vi "Intan_StreamData.vi"(0 "VISA resource name":refnum<visa-resource-name>, 1 "N data blocks to read":i32=1, 5 "refnum in":refnum<file>, 7 "stop":bool, 9 "Save to Disk":bool, 11 "error in":errorcluster, 12 "byte order":T2(ring)=enum."little-endian", 13 "DT_scale":dbl=0.01) -> (2 "Nbytes read":u32, 3 "Nchans1samp_array":u16[](array[numeric]), 4 "Intan Streaming Data  Chart":dbl[][](graph), 6 "path":path, 14 "iteration":i32, 15 "error out":errorcluster)   [LabVIEW 2011]
uses:
  <userlib>/Circular Buffer/Circular Buffer.lvlib
  <userlib>/Circular Buffer/Instance VIs/Circular Buffer(2D I16).vi
  <userlib>/Circular Buffer/Controls/Circular Buffer Operations.ctl
panel:
  out "cluster":T1
  in  "DisplayScale (uV/div)":u16(ring) items=["6400", "3200", "1600", "800", "400", "200", "100", "50", "25"]
  in  "offset factor":dbl=1.0
  out "timestamp":u32[](array[numeric])
  out "'IN' subarray (from INTAN)":u16[](array[numeric])
  in  "start stream (Teensy char)":string="s"
  out "Text response":string
  in  "pause stream (Teensy char)":string="p"
  in  "bytes per block":i32=72
  out "strlen":i32
  out "Nchans":i32
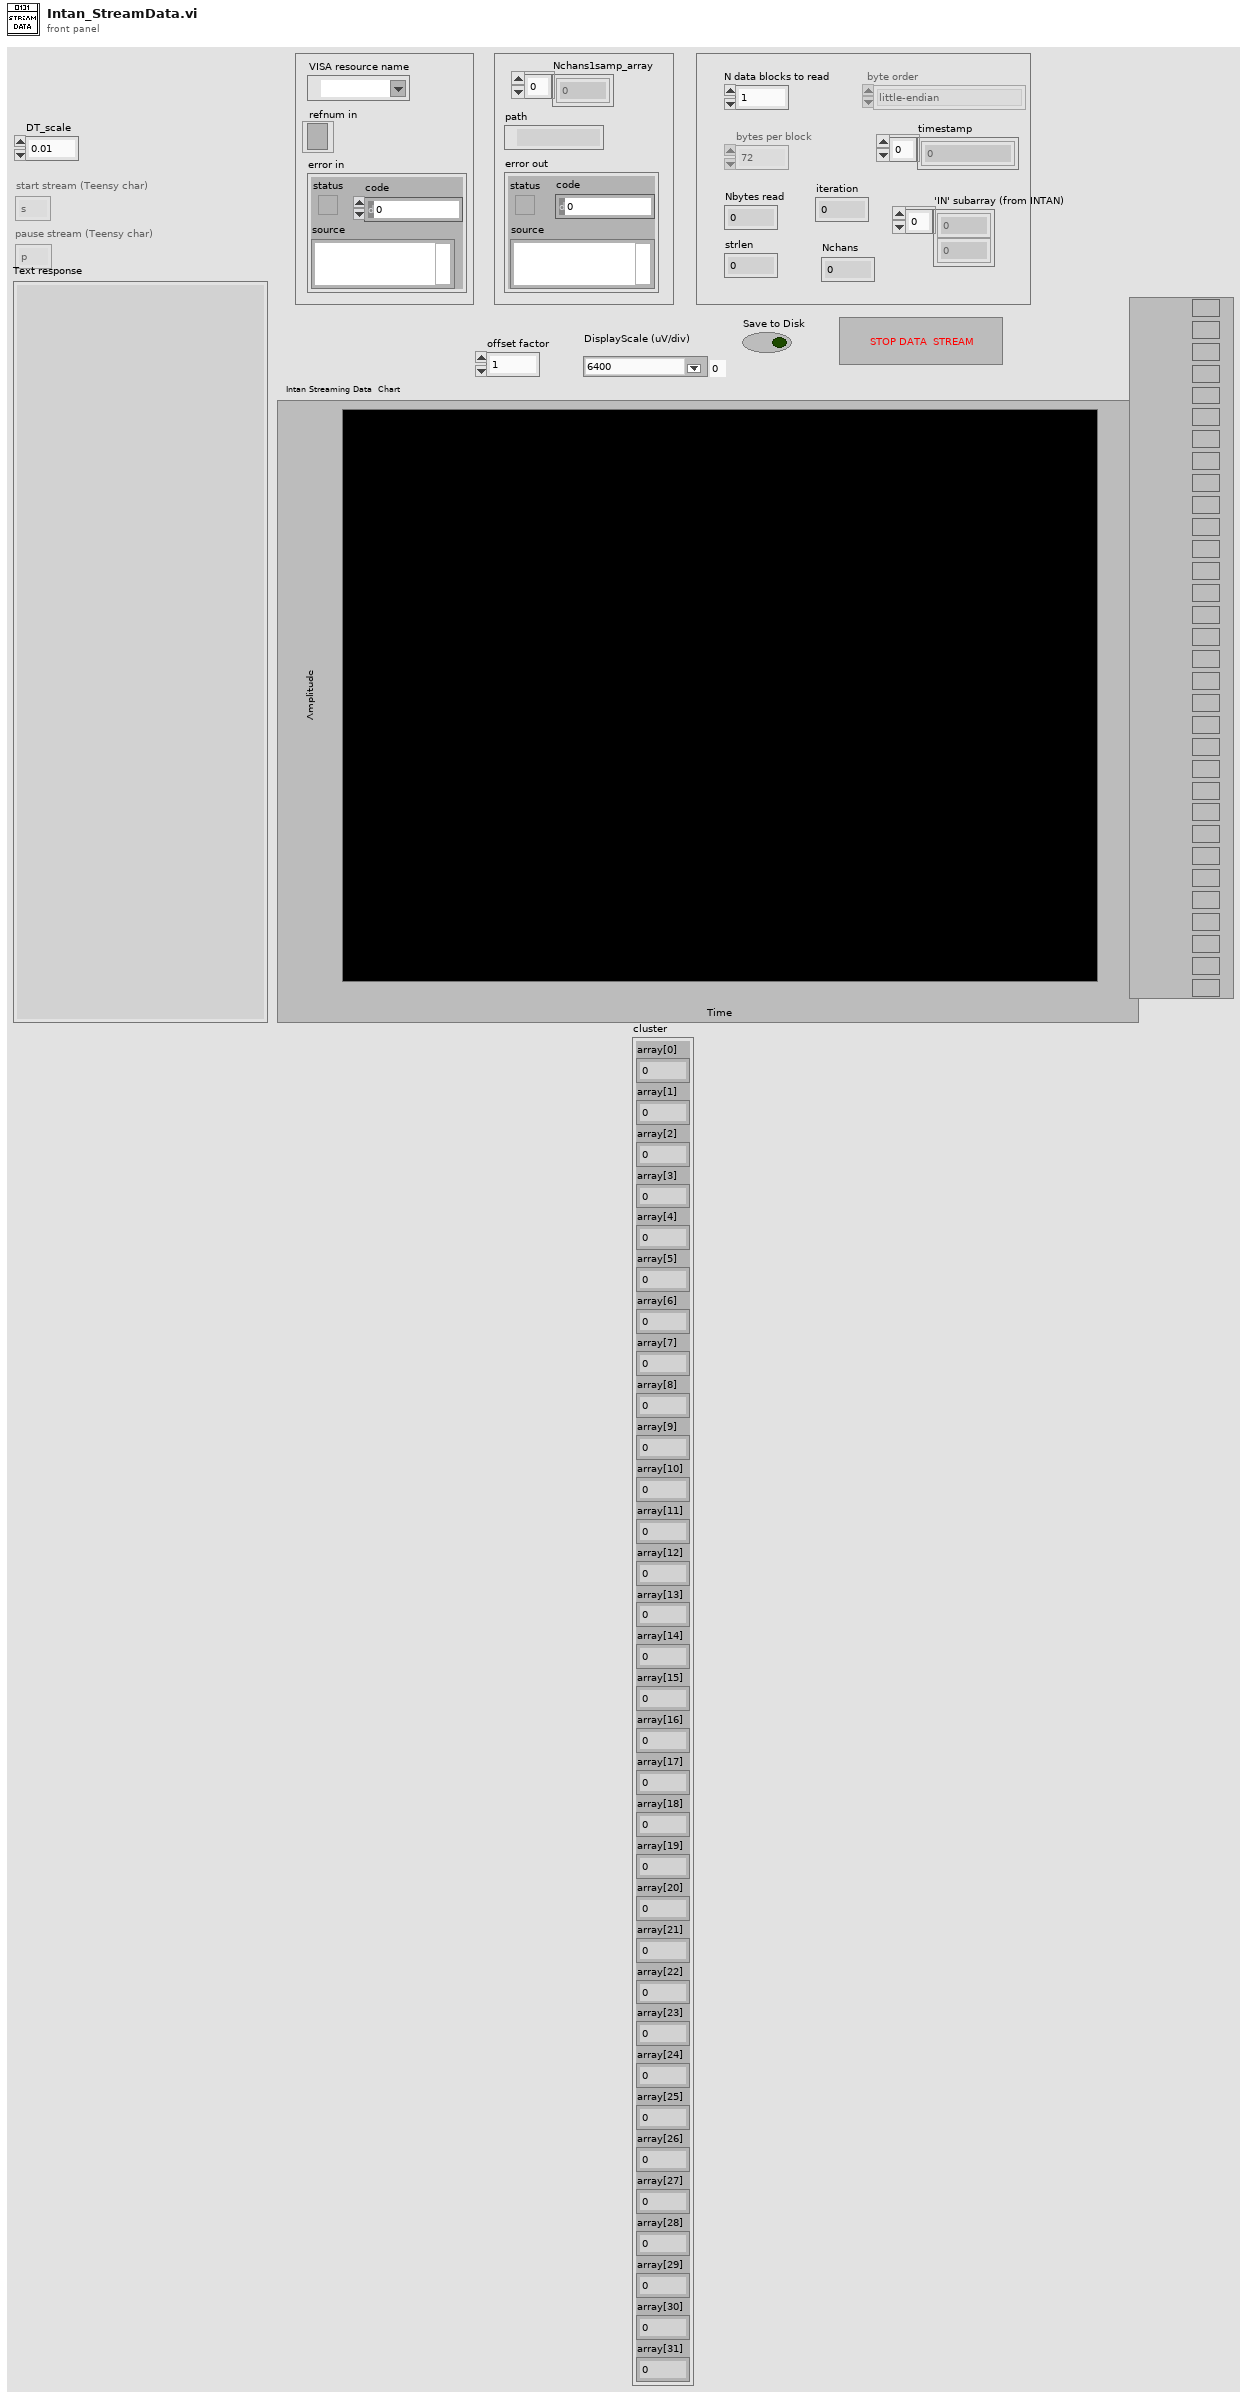
[diagram p1: front panel]
types:
  T1 = cluster{"array[0]":i32, "array[1]":i32, "array[2]":i32, "array[3]":i32, "array[4]":i32, "array[5]":i32, "array[6]":i32, "array[7]":i32, "array[8]":i32, "array[9]":i32, "array[10]":i32, "array[11]":i32, "array[12]":i32, "array[13]":i32, "array[14]":i32, "array[15]":i32, "array[16]":i32, "array[17]":i32, "array[18]":i32, "array[19]":i32, "array[20]":i32, "array[21]":i32, "array[22]":i32, "array[23]":i32, "array[24]":i32, "array[25]":i32, "array[26]":i32, "array[27]":i32, "array[28]":i32, "array[29]":i32, "array[30]":i32, "array[31]":i32}
  T2 = enum16{"big-endian, network order", "native, host order", "little-endian"}
  T3 = cluster{"Samples per Channel":u32, "Channels":u32}
  T4 = typedef "Circular Buffer.lvlib/Circular Buffer Operations.ctl" = enum16{"Initialize", "Get Backlog", "Write", "Read (continuous)", "Read (most recent)"}
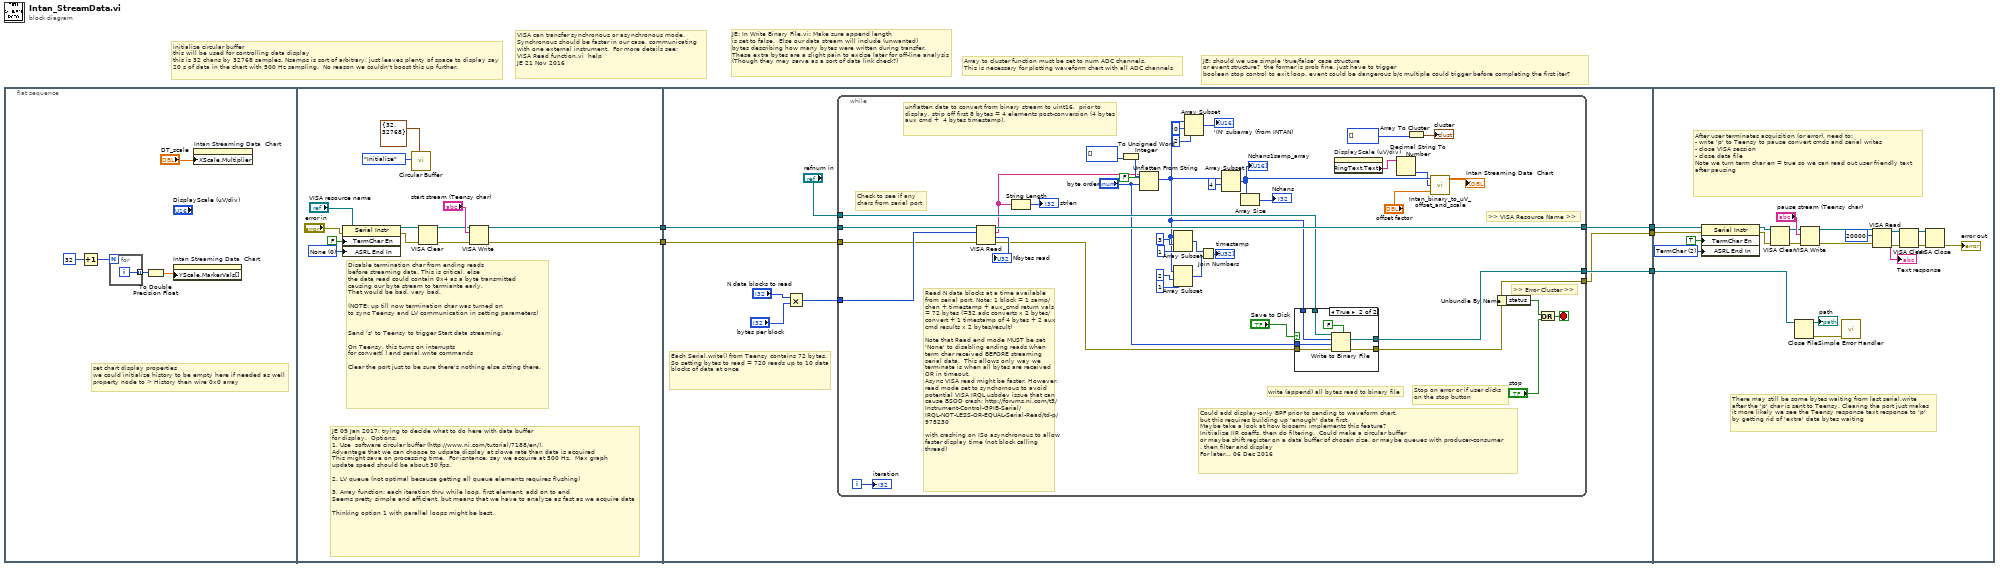
[diagram p0: block diagram]
diagram:
  # "initialize circular buffer\nthis will be used for controlling data display\nthis is 32 chans by 32768 samples. Nsamps is sort of arbitrary, just leaves plenty of space to display say\n20 s of data in the chart with 500 Hz sampling.  No reason we couldn't boost this up further."
  # "JE: should we use simple 'true/false' case structure\nor event structure?  the former is prob fine, just have to trigger\nboolean stop control to exit loop. event could be dangerous b/c multiple could trigger before completing the first iter?"
  # "Array to cluster function must be set to num ADC channels. \nThis is necessary for plotting waveform chart with all ADC channels"
  # "JE: In Write Binary File.vi: Make sure append length \nis set to false.  Else our data stream will include (unwanted)\nbytes describing how many bytes were written during transfer.\nThese extra bytes are a slight pain to excise later for off-line analysis\n(Though they may serve as a sort of data link check?)"
  # "VISA can transfer synchronous or asynchronous mode.\nSynchronous should be faster in our case, communicating\nwith one external instrument.  For more details see: \nVISA Read function.vi  help \nJE 21 Nov 2016"
  n1 = flat-sequence {
    tunnel: [w14] -> w3
    tunnel: [w15] -> w2
    tunnel: [w26] -> w5
    tunnel: [w29] -> w4
    tunnel: w3 -> [w27]
    tunnel: w2 -> [w28]
    tunnel: [w25] -> w1
    tunnel: w5 -> [w87]
    tunnel: w4 -> [w101]
    tunnel: w1 -> [w92]
    frame #0 {
      # "set chart display properties\nwe could initialize history to be empty here if needed as well\nproperty node to > History then wire 0x0 array"
      n2 = Increment(x=32) -> (x+1=w7:i32)
      n3 = for {
        N: w7 -> [_]
        tunnel: [w11] -> w8 mode=indexing
        i -> [w11]
      }
      n4 = To Double Precision Float(number=w8) -> (double precision float=w6:dbl[])
      n5 = property on="Intan Streaming Data  Chart" class="WFChart (strict)"("YScale.MarkerVals[]"=w6) -> ()  [unwired: 2 in, 2 out]
      n6 = property on="Intan Streaming Data  Chart" class="WFChart (strict)"("XScale.Multiplier"="DT_scale") -> ()  [unwired: 2 in, 2 out]
    }
    frame #1 {
      w20 = u16 0 items=["None", "Last Bit", "TermChar"] ("Serial Settings:End Mode for Reads")
      # "JE 09 Jan 2017: trying to decide what to do here with data buffer\nfor display.  Options: \n1. Use  software circular buffer (http://www.ni.com/tutorial/7188/en/). \nAdvantage that we can choose to udpate display at slowe rate than data is acquired\nThis might save on processing time.  For isntance, say we acquire at 500 Hz.  Max graph\nupdate speed should be about 30 fps.\n\n2. LV queue (not optimal because getting all queue elements requires flushing)\n\n3. Array function: each iteration thru while loop, first element, add on to end \nSeems pretty simple and efficient, but means that we have to analyze as fast as we acquire data\n\nThinking option 1 with parallel loops might be best."
      # "Disable termination char from ending reads\nbefore streaming data. This is critical, else\nthe data read could contain 0x4 as a byte transmitted\ncausing our byte stream to termiante early.\nThat would be bad, very bad.\n\n(NOTE: up till now termination char was turned on\nto sync Teensy and LV communication in setting parameters)\n\n\nSend 's' to Teensy to trigger Start data streaming.  \n\nOn Teensy, this turns on interrupts\nfor convert( ) and serial.write commands\n\nClear the port just to be sure there's nothing else sitting there."
      n7 = property class="Serial Instr"(reference="VISA resource name", error in="error in", "TermChar En"=FALSE ("Message Based Settings:Termination Character Enable"), "ASRL End In"=w20) -> (reference out=w19:refnum<visa-resource-name>, error out=w18:errorcluster)
      n8 = call-poly <userlib>:"Circular Buffer.vi"("Buffer Size"=T3 {"Samples per Channel"=32, "Channels"=32768}, "Operation"=Circular_Buffer_Operations."Initialize") -> ()  [unwired: 6 in, 4 out]
      n9 = VISA Clear(VISA resource name=w19, error in (no error)=w18) -> (VISA resource name out=w17:refnum<visa-resource-name>, error out=w16:errorcluster)
      n10 = VISA Write(VISA resource name=w17, write buffer="start stream (Teensy char)", error in (no error)=w16) -> (VISA resource name out=w15:refnum<visa-resource-name>, error out=w14:errorcluster)  [unwired: 1 out]
    }
    frame #2 {
      # "Each Serial.write() from Teensy contains 72 bytes.  So setting bytes to read = 720 reads up to 10 data blocks of data at once"
      n11 = Multiply(x="N data blocks to read", y="bytes per block") -> (x*y=w31:i32)
      n12 = while {
        tunnel: [w72] -> w25
        tunnel: [w73] -> w26
        tunnel: [w68] -> w29
        tunnel: w31 -> [w67]
        tunnel: w27 -> [w63]
        tunnel: "refnum in" -> [w66]
        tunnel: w28 -> [w64]
        i -> [w65]
        stop <- w71 stop-if-true
        # "write (append) all bytes read to binary file"
        # "unflatten data to convert from binary stream to uint16.  prior to display, strip off first 8 bytes = 4 elements post-conversion (4 bytes aux cmd +  4 bytes timestamp)."
        # "Read N data blocks at a time available\nfrom serial port. Note: 1 block = 1 samp/chan + timestamp + aux_cmd return vals = 72 bytes (=32 adc converts x 2 bytes/convert + 1 timestamp of 4 bytes + 2 aux cmd results x 2 bytes/result) \n\nNote that Read end mode MUST be set 'None' to disabling ending reads when term char received BEFORE streaming serial data.  This allows only way we terminate is when all bytes are received OR in timeout.  \nAsync VISA read might be faster. However, read mode set to synchornous to avoid potential VISA IRQL usbdev issue that can cause BSOD crash: http://forums.ni.com/t5/Instrument-Control-GPIB-Serial/IRQL-NOT-LESS-OR-EQUAL-Serial-Read/td-p/975230\n\nwith crashing on ISo asynchronous to allow faster display time (not block calling thread)"
        # "Could add display-only BPF prior to sending to waveform chart.\nbut this requires building up 'enough' data first. \nMaybe take a look at how biosemi implements this feature?\nInitiialize IIR coeffs, then do filtering.  Could make a circular buffer\nor maybe shift register on a data buffer of chosen size, or maybe queues with producer-consumer\n, then filter and display\nFor later... 06 Dec 2016"
        # "Stop on error or if user clicks \non the stop button"
        # ">> Error Cluster >>"
        # ">> VISA Resource Name >>"
        # "Check to see if any\nchars from serial port"
        n13 = VISA Read(VISA resource name=w64, byte count=w67, error in (no error)=w63) -> (VISA resource name out=w73:refnum<visa-resource-name>, read buffer=w53:string, return count=→"Nbytes read":u32, error out=w57:errorcluster)
        n14 = String Length(string=w53) -> (length=→"strlen":i32)
        n15 = To Unsigned Word Integer(number=i16[] []) -> (unsigned 16bit integer=w58:u16[])
        n16 = Unflatten From String(type=w58, binary string=w53, data includes array or string size? (T)=FALSE, byte order (0:big-endian, network order)="byte order") -> (value=w42:u16[])  [unwired: 1 in, 2 out]
        n17 = Array Subset(array=w42, index=3, length=1) -> (w45:u16[])
        n18 = Array Subset(array=w42, index=2, length=1) -> (w44:u16[])
        n19 = Array Subset(array=w42, index=0, length=2) -> (→"'IN' subarray (from INTAN)":u16[])
        n20 = Join Numbers(hi=w45, lo=w44) -> ((hi.lo)=→"timestamp":u32[])
        n21 = Array Subset(array=w42, index=4) -> (w41:u16[])  [unwired: 1 in]
        "Nchans1samp_array" <- w41
        n22 = Array Size(array=w41) -> (size(s)=→"Nchans":i32)
        n23 = case shown="True" "Save to Disk" {
          tunnel: [w75 w82] -> w72
          tunnel: [w74 w81] -> w68
          tunnel: w66 -> [w74 w80]
          tunnel: w57 -> [w75 w79]
          tunnel: "byte order" -> [_ w77]
          tunnel: w42 -> [_ w76]
          frame False {
          }
          frame True {
            n24 = Write to Binary File(file (use dialog)=w80, data=w76, error in=w79, 5:FALSE ("prepend array or string size? (T)"), 9:w77) -> (refnum out=w81:refnum<file>, error out=w82:errorcluster)  [unwired: 1 in, 1 out]
          }
        }
        n25 = property on="DisplayScale (uV/div)" class="Ring (strict)"() -> ("RingText.Text"=w35:string)  [unwired: 2 in, 2 out]
        n26 = Decimal String To Number(string=w35) -> (number=w34:i32)  [unwired: 2 in, 1 out]
        n27 = Array To Cluster(array=i32[] []) -> (cluster=→"cluster":T1)
        n28 = call "Intan_binary_to_uV_offset_and_scale.vi"("offset spacing factor"="offset factor", "Yscale (uv/div)"=w34, "BinaryData [Nchans x Nsamps]"=w41) -> ("Data4Display"=→"Intan Streaming Data  Chart":dbl[][])  [unwired: 1 in, 1 out]
        n29 = Unbundle By Name(w72) -> ("status"=w70:bool)
        n30 = Or(x=w70, y="stop") -> (x .or. y?=w71:bool)
        "iteration" <- w65
      }
    }
    frame #3 {
      w93 = u16 2 items=["None", "Last Bit", "TermChar"] ("Serial Settings:End Mode for Reads")
      # "There may still be some bytes waiting from last serial.write\nafter the 'p' char is sent to Teensy. Clearing the port just makes\nit more likely we see the Teensy response text response to 'p' \nby getting rid of 'extra' data bytes waiting"
      # "After user terminates acquisition (or error), need to:\n- write 'p' to Teensy to pause convert cmds and serial writes\n- close VISA session\n- close data file\nNote we turn term char en = true so we can read out user friendly text \nafter pausing"
      n31 = property class="Serial Instr"(reference=w87, error in=w92, "TermChar En"=TRUE ("Message Based Settings:Termination Character Enable"), "ASRL End In"=w93) -> (reference out=w86:refnum<visa-resource-name>, error out=w85:errorcluster)
      n32 = VISA Clear(VISA resource name=w86, error in (no error)=w85) -> (VISA resource name out=w84:refnum<visa-resource-name>, error out=w83:errorcluster)
      n33 = Close File(refnum=w101) -> (path=→"path":path, error out=w102:errorcluster)  [unwired: 1 in]
      n34 = VISA Write(VISA resource name=w84, write buffer="pause stream (Teensy char)", error in (no error)=w83) -> (VISA resource name out=w96:refnum<visa-resource-name>, error out=w95:errorcluster)  [unwired: 1 out]
      n35 = call <vilib>:"Simple Error Handler.vi"("error in (no error)"=w102) -> ()  [unwired: 4 in, 5 out]
      n36 = VISA Read(VISA resource name=w96, byte count=u32 20000, error in (no error)=w95) -> (VISA resource name out=w91:refnum<visa-resource-name>, read buffer=→"Text response":string, error out=w89:errorcluster)  [unwired: 1 out]
      n37 = VISA Clear(VISA resource name=w91, error in (no error)=w89) -> (VISA resource name out=w90:refnum<visa-resource-name>, error out=w88:errorcluster)
      n38 = VISA Close(VISA resource name=w90, error in (no error)=w88) -> (error out=→"error out":errorcluster)
    }
  }
